vi "dataFromBooleanArray.vi"(1 "Boolean array":bool[](array[boolean])) -> (0 "Data":u8[](array[numeric]))   [LabVIEW 2017, in "canopen.lvlib"]
doc: "Converts an array of booleans to its binary data representation."
uses:
  canopen.lvlib
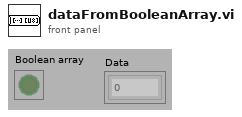
[diagram p1: front panel]
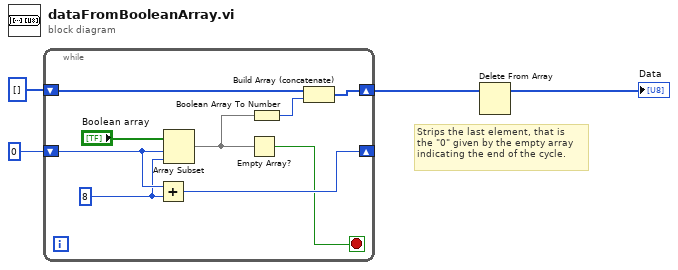
[diagram p0: block diagram]
diagram:
  # "Strips the last element, that is\nthe \"0\" given by the empty array\nindicating the end of the cycle."
  n1 = while {
    shift-right: [w11] -> w2
    shift-left: u8[] [] ("Data") -> [w12]
    shift-right: [w8] -> _
    shift-left: 0 ("index") -> [w9]
    stop <- w6 stop-if-true
    w5 = 8 ("y")
    n2 = Add(x=w9, y=w5) -> (x+y=w8:i32)
    n3 = Array Subset(array="Boolean array", index=w9, length=w5) -> (w7:bool[])
    n4 = Empty Array?(array=w7) -> (empty?=w6:bool)
    n5 = Boolean Array To Number(Boolean array=w7) -> (number=w13:u8)
    n6 = Build Array (concatenate)(w12, w13) -> (w11:u8[])
  }
  n7 = Delete From Array(array=w2) -> (array with subset deleted=→"Data":u8[])  [unwired: 2 in, 1 out]
